vi "QiG_UI_Simple.vi"() -> ()   [LabVIEW 2010]
uses:
  TS Simple LabVIEW OI Dependencies.lvlib
panel:
  in  "Terminate All Button":refnum<k7>(container)
  in  "Exit Button":refnum<k7>(container)
  in  "Login/Logout Button":refnum<k7>(container)
  in  "Close Executions Button":refnum<k7>(container)
  in  "Break/Resume Button":refnum<k7>(container)
  in  "Terminate/Restart Button":refnum<k7>(container)
  in  "Run Selected Sequence Button":refnum<k7>(container)
  in  "Entry Point 2 Button":refnum<k7>(container)
  in  "Entry Point 1 Button":refnum<k7>(container)
  in  "Report Viewer":refnum<k7>(container)
  in  "Close Sequence File Button":refnum<k7>(container)
  in  "Open Sequence File Button":refnum<k7>(container)
  in  "Executions ComboBox":refnum<k7>(container) caption="Executions:"
  in  "Sequences ComboBox":refnum<k7>(container) caption="Sequences:"
  in  "Execution View":refnum<k7>(container)
  in  "Sequence Files ComboBox":refnum<k7>(container) caption="Sequence File:"
  in  "ExecutionView Manager":refnum<k7>(container)
  in  "SequenceFileView Manager":refnum<k7>(container)
  in  "Application Manager":refnum<k7>(container)
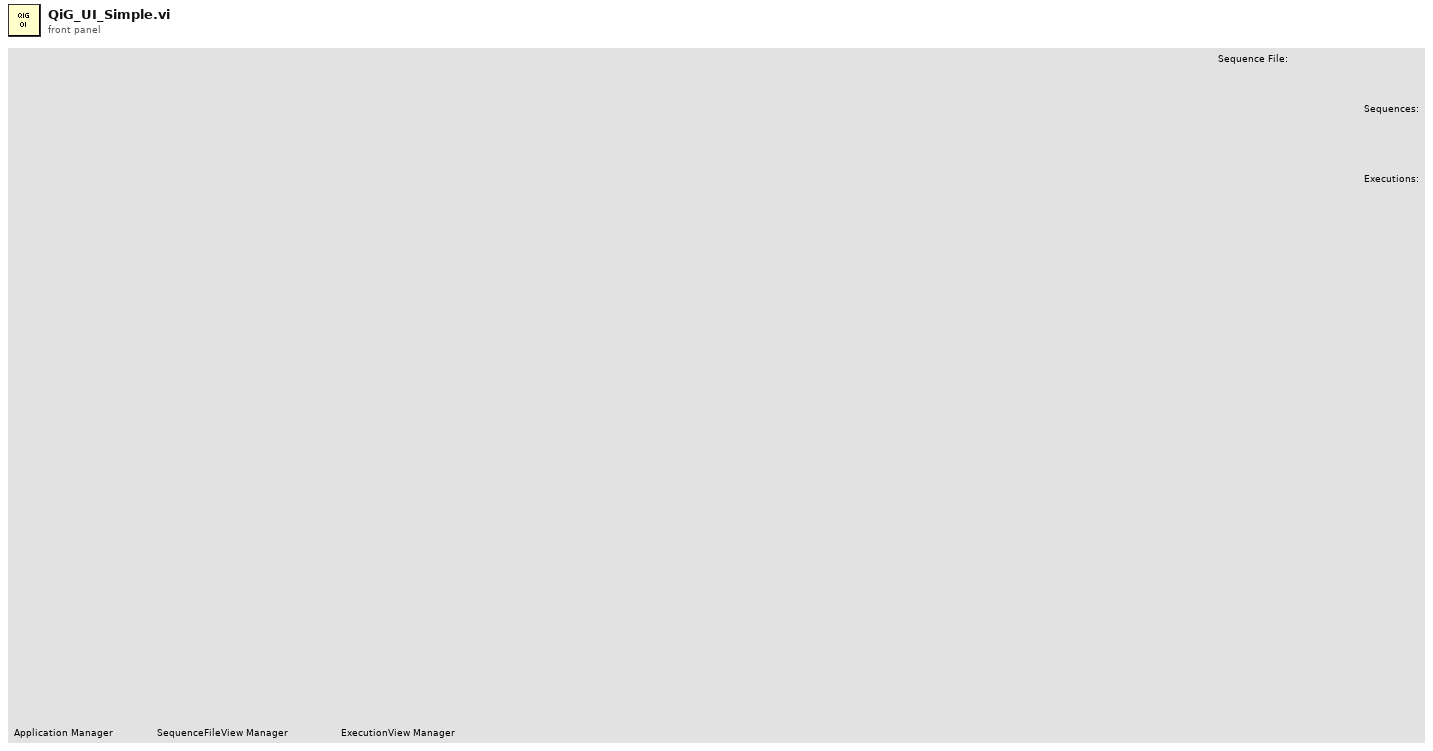
[diagram p1: front panel]
types:
  T1 = enum16{"Default Sequence", "Board Test Sequence"}
  T2 = enum32{"invalid app kind", "Development System", "Run Time System", "Student Edition", "Embedded LabVIEW", "Evaluation", "Custom"}
  T3 = cluster{"Login/Logout Button":refnum<k7>, "Exit Button":refnum<k7>, "Terminate All Button":refnum<k7>}
  T4 = cluster{"Sequence Files ComboBox":refnum<k7>, "Sequences ComboBox":refnum<k7>, "Open Sequence File Button":refnum<k7>, "Close Sequence File Button":refnum<k7>, "Entry Point 1 Button":refnum<k7>, "Entry Point 2 Button":refnum<k7>, "Run Selected Sequence Button":refnum<k7>}
  T5 = cluster{"Executions ComboBox":refnum<k7>, "Execution View":refnum<k7>, "Report Viewer":refnum<k7>, "Close Executions Button":refnum<k7>, "Break/Resume Button":refnum<k7>, "Terminate/Restart Button":refnum<k7>}
  T6 = cluster{"Quit Application Event":refnum<user-event>, refnum<vi>, "ExecutionView Manager":refnum<k7>, "SequenceFileView Manager":refnum<k7>}
  T7 = enum8{"Enabled", "Disabled", "Disabled and Grayed Out"}
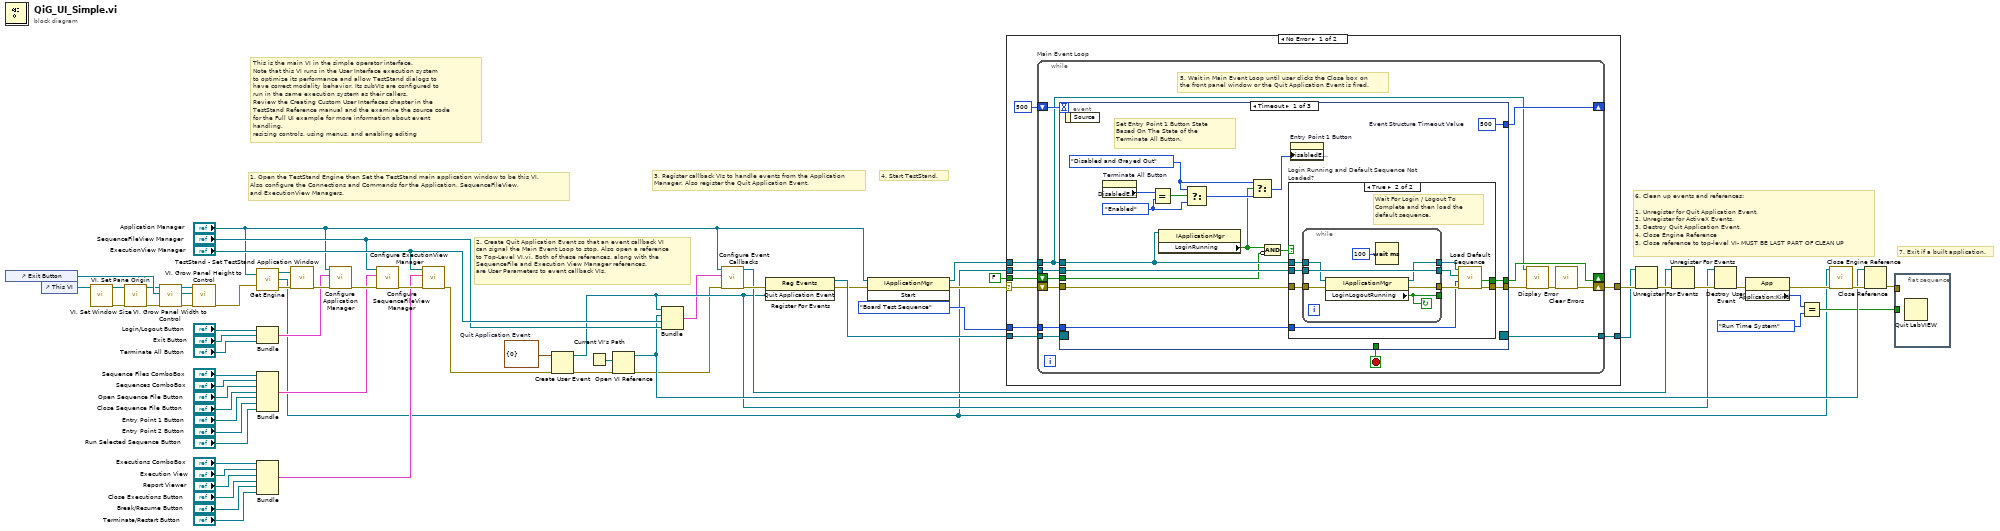
[diagram p0: block diagram]
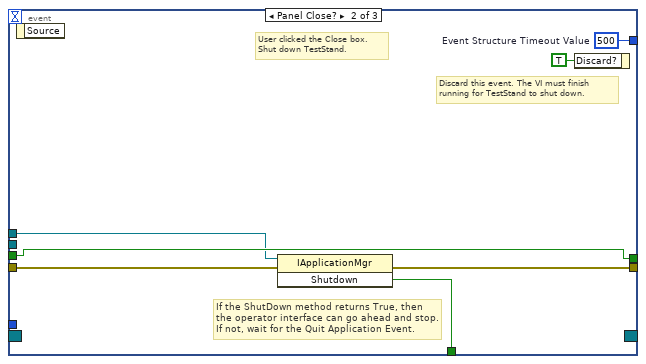
[diagram p3: hidden frame]
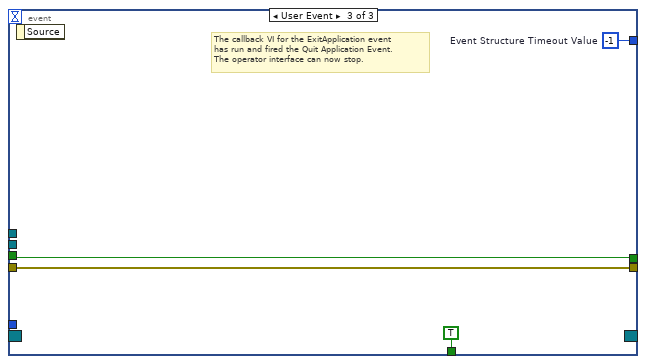
[diagram p4: hidden frame]
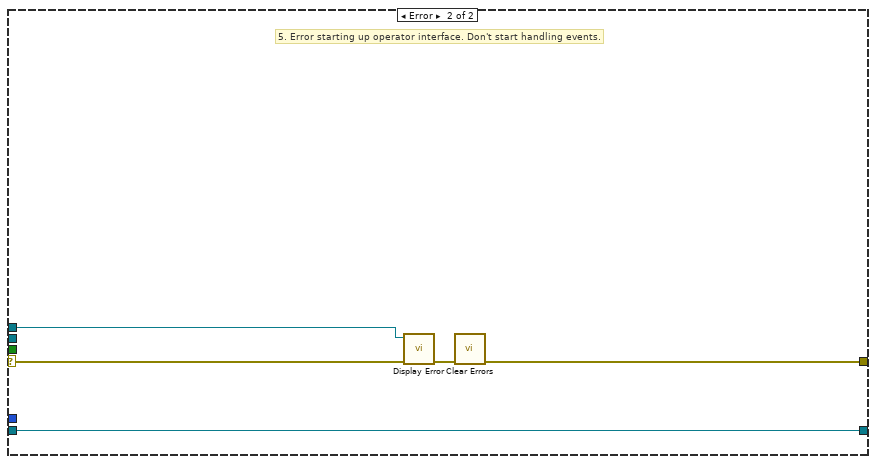
[diagram p5: hidden frame]
diagram:
  w59 = cluster{"Number":i32} {"Number"=0}  # Quit Application Event
  # "This is the main VI in the simple operator interface.\nNote that this VI runs in the User Interface execution system\nto optimize its performance and allow TestStand dialogs to\nhave correct modality behavior. Its subVIs are configured to\nrun in the same execution system as their callers.\nReview the Creating Custom User Interfaces chapter in the \nTestStand Reference manual and the examine the source code\nfor the Full UI example for more information about event handling,\nresizing controls, using menus, and enabling editing"
  # "7. Exit if a built application."
  # "4. Start TestStand."
  # "3. Register callback VIs to handle events from the Application\nManager. Also register the Quit Application Event."
  # "2. Create Quit Application Event so that an event callback VI\ncan signal the Main Event Loop to stop. Also open a reference\nto Top-Level VI.vi. Both of these references, along with the\nSequenceFile and Execution View Manager references,\nare User Parameters to event callback VIs."
  # "6. Clean up events and references:\n\n1. Unregister for Quit Application Event.\n2. Unregister for ActiveX Events.\n3. Destroy Quit Application Event.\n4. Close Engine Reference\n5. Close reference to top-level VI- MUST BE LAST PART OF CLEAN UP"
  # "1. Open the TestStand Engine then Set the TestStand main application window to be this VI. \nAlso configure the Connections and Commands for the Application, SequenceFileView, \nand ExecutionView Managers."
  n1 = control-ref of="Exit Button"() -> (w7:refnum<vi>)
  n2 = control-ref of="This VI"() -> (w3:refnum<vi>)
  n3 = call "VI, Set Window Size.vi"("VI ref"=w3) -> ("error out"=w2:errorcluster, "VI ref dup"=w1:refnum<vi>)  [unwired: 7 in]
  n4 = call "VI, Set Pane Origin.vi"("error in"=w2, "VI ref"=w1) -> ("error out"=w5:errorcluster, "VI ref dup"=w4:refnum<vi>)  [unwired: 6 in]
  n5 = call "VI, Grow Panel Width to Control.vi"("error in"=w5, "Ctl ref"=w7, "VI ref"=w4) -> ("error out"=w10:errorcluster, "Ctl ref dup"=w8:refnum<vi>, "VI ref dup"=w9:refnum<vi>)  [unwired: 4 in]
  n6 = call "VI, Grow Panel Height to Control.vi"("error in"=w10, "Ctl ref"=w8, "VI ref"=w9) -> ("error out"=w6:errorcluster)  [unwired: 4 in, 2 out]
  n7 = call "Get Engine.vi"("Application Manager In"="Application Manager", "error in (no error)"=w6) -> ("Application Manager Out"=w21:refnum<k7>, "TestStand Engine"=w13:refnum<k7>, "error out"=w22:errorcluster)
  n8 = Bundle("Login/Logout Button"="Login/Logout Button", "Exit Button"="Exit Button", "Terminate All Button"="Terminate All Button") -> (w31:T3)  [unwired: 1 out]
  n9 = Bundle("Sequence Files ComboBox"="Sequence Files ComboBox", "Sequences ComboBox"="Sequences ComboBox", "Open Sequence File Button"="Open Sequence File Button", "Close Sequence File Button"="Close Sequence File Button", "Entry Point 1 Button"="Entry Point 1 Button", "Entry Point 2 Button"="Entry Point 2 Button", "Run Selected Sequence Button"="Run Selected Sequence Button") -> (w26:T4)  [unwired: 1 out]
  n10 = Bundle("Executions ComboBox"="Executions ComboBox", "Execution View"="Execution View", "Report Viewer"="Report Viewer", "Close Executions Button"="Close Executions Button", "Break/Resume Button"="Break/Resume Button", "Terminate/Restart Button"="Terminate/Restart Button") -> (w42:T5)  [unwired: 1 out]
  n11 = call <vilib>:"TestStand - Set TestStand Application Window.vi"("error in (no error)"=w22, "Application Manager"=w21) -> ("error out"=w65:errorcluster)  [unwired: 1 in, 8 out]
  n12 = call "Configure Application Manager.vi"("error in (no error)"=w65, "UI Control References"=w31, "Application Manager"="Application Manager") -> ("error out"=w34:errorcluster)  [unwired: 8 out]
  n13 = call "Configure SequenceFileView Manager.vi"("error in (no error)"=w34, "UI Control References"=w26, "SequenceFileView Manager"="SequenceFileView Manager") -> ("error out"=w64:errorcluster)  [unwired: 7 in, 1 out]
  n14 = call "Configure ExecutionView Manager.vi"("error in (no error)"=w64, "UI Control References"=w42, "ExecutionView Manager"="ExecutionView Manager") -> ("error out"=w23:errorcluster)  [unwired: 5 in, 3 out]
  n15 = Create User Event(user event datatype=w59, error in=w23) -> (user event=w35:refnum<user-event>, error out=w40:errorcluster)
  n16 = Current VI's Path() -> (path=w58:path)
  n17 = Open VI Reference(vi path=w58, error in (no error)=w40) -> (vi reference=w36:refnum<vi>, error out=w17:errorcluster)  [unwired: 4 out]
  n18 = Bundle("Quit Application Event"=w35, w36, "ExecutionView Manager"="ExecutionView Manager", "SequenceFileView Manager"="SequenceFileView Manager") -> (w18:T6)  [unwired: 1 out]
  n19 = call "Configure Event Callbacks.vi"("error in (no error)"=w17, "User Parameters"=w18, "Application Manager"="Application Manager") -> ("error out"=w39:errorcluster, "Event Callback Refnum Out"=w37:refnum<k27>)  [unwired: 4 in, 3 out]
  n20 = register-events(error in=w39, w35) -> (reference out=w60:refnum<event-registration>, error out=w11:errorcluster)  [unwired: 1 in]
  n21 = invoke class="IApplicationMgr" method="Start"(reference="Application Manager", error in=w11) -> (reference out=w12:refnum<k7>, error out=w14:errorcluster)  [unwired: 1 in, 1 out]
  n22 = case shown="No Error" w14 {
    selector: w14 -> [w71 w136]
    tunnel: w60 -> [w74 w138]
    tunnel: [w73 w138] -> w57
    tunnel: w12 -> [w72 w135]
    tunnel: [w70 w137] -> w62
    tunnel: T1."Board Test Sequence" ("Select Sequence to Load") -> [w69 _]
    tunnel: w13 -> [w68 _]
    tunnel: FALSE ("Loaded?") -> [w66 _]
    frame No Error {
      n23 = while "Main Event Loop" {
        tunnel: w74 -> [w84]
        tunnel: [w83] -> w73
        shift-right: [w79] -> w70
        shift-left: w71 -> [w82]
        tunnel: w72 -> [w78]
        tunnel: w69 -> [w77]
        tunnel: w68 -> [w76]
        shift-right: [w88] -> _
        shift-left: 500 -> [w86]
        shift-right: [w87] -> _
        shift-left: w66 -> [w75]
        stop <- w85 stop-if-true
        # "5. Wait in Main Event Loop until user clicks the Close box on\nthe front panel window or the Quit Application Event is fired."
        n24 = event shown="[0] Timeout" {
          selector: w84 -> [_ _ _]
          dyn-events: [_ _ _] -> w83
          timeout: w86 -> [_ _ _]
          tunnel: w78 -> [w99 w123 _]
          tunnel: w82 -> [w101 w129 w131]
          tunnel: [_ w128 TRUE ("ShutDown")] -> w85
          tunnel: [w104 w127 w131] -> w81
          tunnel: w77 -> [w103 _ _]
          tunnel: w76 -> [w100 _ _]
          tunnel: [w102 w125 w132] -> w88
          tunnel: w75 -> [w93 w124 w130]
          tunnel: [w98 w124 w130] -> w87
          event Timeout {
            w96 = T7."Enabled" ("y")
            w90 = T7."Disabled and Grayed Out" ("y")
            w102 = 500  # Event Structure Timeout Value
            # "Set Entry Point 1 Button State Based On The State of the Terminate All Button."
            n25 = event-data() -> ()  [unwired: 2 out]
            n26 = property on="Terminate All Button" class="AXCont"() -> ("DisabledEnum"=w97:T7)  [unwired: 2 in, 2 out]
            n27 = Equal?(x=w97, y=w96) -> (x = y?=w95:bool)
            n28 = property class="IApplicationMgr"(reference=w99) -> ("LoginRunning"=w91:bool)  [unwired: 1 in, 2 out]
            n29 = Select(t=w90, s=w95, f=w96) -> (s? t:f=w92:T7)
            n30 = Select(t=w90, s=w91, f=w92) -> (s? t:f=w89:T7)
            n31 = Compound Arithmetic op=AND(w91, invert w93) -> (w94:bool)
            n32 = case "Login Running and Default Sequence Not Loaded?" shown="True" w94 {
              selector: w94 -> [w105 _]
              tunnel: [w106 w114] -> w104
              tunnel: w103 -> [_ w113]
              tunnel: w101 -> [w106 w111]
              tunnel: w100 -> [_ w108]
              tunnel: w99 -> [_ w110]
              tunnel: [w105 w112] -> w98
              frame False {
                # "Login Not Running or Default Sequence is Already Loaded. Do Not Load The Default Sequence."
              }
              frame True {
                # "Wait For Login / Logout To Complete and then load the default sequence."
                n33 = while {
                  tunnel: [w121] -> _
                  tunnel: w110 -> [w120]
                  tunnel: w111 -> [w119]
                  tunnel: [w118] -> w115
                  tunnel: [w117] -> w109
                  tunnel: w108 -> [w122]
                  tunnel: [w122] -> w107
                  stop <- w121 continue-if-true
                  n34 = property class="IApplicationMgr"(reference=w120, error in=w119) -> (reference out=w117:refnum<k7>, error out=w118:errorcluster, "LoginLogoutRunning"=w121:bool)
                  n35 = Wait (ms)(milliseconds to wait=u32 100) -> ()  [unwired: 1 out]
                }
                n36 = call "Load Default Sequence.vi"("error in"=w115, "Select Sequence to Load"=w113, "TestStand Engine"=w107, "Application Manager"=w109) -> ("error out"=w114:errorcluster, "Loaded?"=w112:bool)  [unwired: 4 in, 2 out]
              }
            }
            n37 = property on="Entry Point 1 Button" class="AXCont"("DisabledEnum"=w89) -> ()  [unwired: 2 in, 2 out]
          }
          event Panel Close? {
            w125 = 500  # Event Structure Timeout Value
            # "Discard this event. The VI must finish\nrunning for TestStand to shut down."
            # "If the ShutDown method returns True, then\nthe operator interface can go ahead and stop.\nIf not, wait for the Quit Application Event."
            # "User clicked the Close box.\nShut down TestStand."
            n38 = event-data() -> ()  [unwired: 2 out]
            n39 = invoke class="IApplicationMgr" method="Shutdown"(reference=w123, error in=w129) -> (error out=w127:errorcluster, "Shutdown"=w128:bool)  [unwired: 1 in, 1 out]
            n40 = event-data("Discard?"=TRUE) -> ()  [unwired: 1 in, 1 out]
          }
          event User Event {
            w132 = -1  # Event Structure Timeout Value
            # "The callback VI for the ExitApplication event\nhas run and fired the Quit Application Event.\nThe operator interface can now stop."
            n41 = event-data() -> ()  [unwired: 2 out]
          }
        }
        n42 = call "Display Error.vi"("error in (no error)"=w81, "Application Manager"=w78) -> ("error out"=w80:errorcluster)  [unwired: 9 out]
        n43 = call <vilib>:"Clear Errors.vi"("error in (no error)"=w80) -> ("error out"=w79:errorcluster)  [unwired: 6 out]
      }
    }
    frame Error {
      # "5. Error starting up operator interface. Don't start handling events."
      n44 = call "Display Error.vi"("error in (no error)"=w136, "Application Manager"=w135) -> ("error out"=w134:errorcluster)  [unwired: 9 out]
      n45 = call <vilib>:"Clear Errors.vi"("error in (no error)"=w134) -> ("error out"=w137:errorcluster)  [unwired: 6 out]
    }
  }
  n46 = Unregister For Events(event registration refnum=w57, error in=w62) -> (error out=w56:errorcluster)
  n47 = Unregister For Events(event registration refnum=w37, error in=w56) -> (error out=w61:errorcluster)
  n48 = Destroy User Event(user event=w35, error in=w61) -> (error out=w30:errorcluster)
  n49 = property class="App"(error in=w30) -> (error out=w20:errorcluster, "Application:Kind"=w29:T2)  [unwired: 1 in, 1 out]
  n50 = Equal?(x=w29, y=T2."Run Time System" ("Application:Kind")) -> (x = y?=w27:bool)
  n51 = call "Close Engine Reference.vi"("error in (no error)"=w20, "TestStand Engine"=w13) -> ("error out"=w63:errorcluster)  [unwired: 1 in, 8 out]
  n52 = Close Reference(reference=w36, error in (no error)=w63) -> (error out=w24:errorcluster)
  n53 = flat-sequence {
    tunnel: w27 -> [_]
    tunnel: w24 -> [_]
    frame #0 {
      n54 = Quit LabVIEW() -> ()  [unwired: 1 in]
    }
  }
